vi "Create Arbitrary 111 Twin.vi"(10 "Additional Strain/twin (A)":dbl(slide) scale=0.0..10.0, 11 "Periodicity":i32[](array[numeric])=[3, 3]) -> (2 "# of extra cells needed for cubic":i32, 3 "AnBm Twin":T1={"Structure Name"="111 Twin, A6B1A4B1", "Lattice vector a"=[4.67354, 0.0, 0.0], "Lattice vector b"=[0.0, 8.0948, 0.0], "Lattice vector c"=[0.0, 0.0, 45.791158], "Atoms Array"=[{"Atom Name"="Cd", "Positions (Direct)"=[[0.0, 0.333334, 0.02083326728856693], [0.500001, 0.833335, 0.02083326728856693], [0.500001, 0.166667, 0.10416683644324957], [0.0, 0.666668, 0.10416683644324957], [0.0, 0.0, 0.18750008462334786], [0.500001, 0.500001, 0.18750008462334786], [0.0, 0.333334, 0.2708334092373685], [0.500001, 0.833335, 0.2708334092373685], [0.500001, 0.166667, 0.35416697839205113], [0.0, 0.666668, 0.35416697839205113], [0.0, 0.0, 0.4375002265721494], [0.500001, 0.500001, 0.4375002265721494], [0.500001, 0.166667, 0.5208335530060322], [0.0, 0.666668, 0.5208335530060322], [0.0, 0.0, 0.6041666821354701], [0.500001, 0.500001, 0.6041666821354701], [0.0, 0.333334, 0.6875000067494909], [0.500001, 0.833335, 0.6875000067494909], [0.500001, 0.166667, 0.7708335759041735], [0.0, 0.666668, 0.7708335759041735], [0.0, 0.0, 0.8541668240842718], [0.500001, 0.500001, 0.8541668240842718], [0.500001, 0.166667, 0.9375001505181546], [0.0, 0.666668, 0.9375001505181546]], "Positions (Cartesian)"=[[0.0, 2.6982720632, 0.9539794340669999], [2.3367746735400003, 6.745680158, 0.9539794340669999], [2.3367746735400003, 1.3491360316, 4.769920065932999], [0.0, 5.3965441264, 4.769920065932999], [0.0, 0.0, 8.585846000001093], [2.3367746735400003, 4.0474080948, 8.585846000001093], [0.0, 2.6982720632, 12.401775434067], [2.3367746735400003, 6.745680158, 12.401775434067], [2.3367746735400003, 1.3491360316, 16.217716065933], [0.0, 5.3965441264, 16.217716065933], [0.0, 0.0, 20.03364200000109], [2.3367746735400003, 4.0474080948, 20.03364200000109], [2.3367746735400003, 1.3491360316, 23.849571517400598], [0.0, 5.3965441264, 23.849571517400598], [0.0, 0.0, 27.66549200000109], [2.3367746735400003, 4.0474080948, 27.66549200000109], [0.0, 2.6982720632, 31.481421434067002], [2.3367746735400003, 6.745680158, 31.481421434067002], [2.3367746735400003, 1.3491360316, 35.297362065933], [0.0, 5.3965441264, 35.297362065933], [0.0, 0.0, 39.1132880000011], [2.3367746735400003, 4.0474080948, 39.1132880000011], [2.3367746735400003, 1.3491360316, 42.9292175174006], [0.0, 5.3965441264, 42.9292175174006]]}, {"Atom Name"="Te", "Positions (Direct)"=[[0.0, 0.0, 0.0], [0.500001, 0.500001, 0.0], [0.0, 0.333334, 0.08333356915468265], [0.500001, 0.833335, 0.08333356915468265], [0.500001, 0.166667, 0.16666681551492246], [0.0, 0.666668, 0.16666681551492246], [0.0, 0.0, 0.25000014194880155], [0.500001, 0.500001, 0.25000014194880155], [0.0, 0.333334, 0.3333337111034842], [0.500001, 0.833335, 0.3333337111034842], [0.500001, 0.166667, 0.41666695746372406], [0.0, 0.666668, 0.41666695746372406], [0.0, 0.0, 0.5000002838976031], [0.500001, 0.500001, 0.5000002838976031], [0.500001, 0.166667, 0.5833334130270448], [0.0, 0.666668, 0.5833334130270448], [0.0, 0.0, 0.6666667394609238], [0.500001, 0.500001, 0.6666667394609238], [0.0, 0.333334, 0.7500003086156065], [0.500001, 0.833335, 0.7500003086156065], [0.500001, 0.166667, 0.8333335549758464], [0.0, 0.666668, 0.8333335549758464], [0.0, 0.0, 0.9166668814097255], [0.500001, 0.500001, 0.9166668814097255]], "Positions (Cartesian)"=[[0.0, 0.0, 0.0], [2.3367746735400003, 4.0474080948, 0.0], [0.0, 2.6982720632, 3.815940631866], [2.3367746735400003, 6.745680158, 3.815940631866], [2.3367746735400003, 1.3491360316, 7.631866482600667], [0.0, 5.3965441264, 7.631866482600667], [0.0, 0.0, 11.447796], [2.3367746735400003, 4.0474080948, 11.447796], [0.0, 2.6982720632, 15.263736631866], [2.3367746735400003, 6.745680158, 15.263736631866], [2.3367746735400003, 1.3491360316, 19.079662482600668], [0.0, 5.3965441264, 19.079662482600668], [0.0, 0.0, 22.895592], [2.3367746735400003, 4.0474080948, 22.895592], [2.3367746735400003, 1.3491360316, 26.711512482600668], [0.0, 5.3965441264, 26.711512482600668], [0.0, 0.0, 30.527442], [2.3367746735400003, 4.0474080948, 30.527442], [0.0, 2.6982720632, 34.343382631866], [2.3367746735400003, 6.745680158, 34.343382631866], [2.3367746735400003, 1.3491360316, 38.15930848260067], [0.0, 5.3965441264, 38.15930848260067], [0.0, 0.0, 41.975238000000004], [2.3367746735400003, 4.0474080948, 41.975238000000004]]}], "# of atoms"=48})   [LabVIEW 2010]
uses:
  <vilib>/Analysis/baseanly.llb/A x Vector.vi
  <vilib>/Analysis/NI_AALBase.lvlib
panel:
  in  "Twins":T2(array[cluster])=[{"Structure Name"="111", "Lattice vector a"=[4.67354, 0.0, 0.0], "Lattice vector b"=[0.0, 8.0948, 0.0], "Lattice vector c"=[0.0, 0.0, 3.81592], "Atoms Array"=[{"Atom Name"="Cd", "Positions (Direct)"=[[0.500001, 0.166667, 0.24999987353], [0.0, 0.666668, 0.24999987353]], "Positions (Cartesian)"=[[2.3367746735400003, 1.3491360316, 0.9539795174005976], [0.0, 5.3965441264, 0.9539795174005976]]}, {"Atom Name"="Te", "Positions (Direct)"=[[0.0, 0.0, 0.0], [0.500001, 0.500001, 0.0]], "Positions (Cartesian)"=[[0.0, 0.0, 0.0], [2.3367746735400003, 4.0474080948, 0.0]]}], "# of atoms"=4}, {"Structure Name"="111", "Lattice vector a"=[4.67354, 0.0, 0.0], "Lattice vector b"=[0.0, 8.0948, 0.0], "Lattice vector c"=[0.0, 0.0, 3.81595], "Atoms Array"=[{"Atom Name"="Cd", "Positions (Direct)"=[[0.0, 0.333334, 0.250000402207], [0.500001, 0.833335, 0.250000402207]], "Positions (Cartesian)"=[[0.0, 2.6982720632, 0.9539890348018015], [2.3367746735400003, 6.745680158, 0.9539890348018015]]}, {"Atom Name"="Te", "Positions (Direct)"=[[0.500001, 0.166667, 2.49411e-06], [0.0, 0.666668, 2.49411e-06]], "Positions (Cartesian)"=[[2.3367746735400003, 1.3491360316, 9.5173990545e-06], [0.0, 5.3965441264, 9.5173990545e-06]]}], "# of atoms"=4}, {"Structure Name"="111", "Lattice vector a"=[4.67354, 0.0, 0.0], "Lattice vector b"=[0.0, 8.0948, 0.0], "Lattice vector c"=[0.0, 0.0, 3.81593], "Atoms Array"=[{"Atom Name"="Cd", "Positions (Direct)"=[[0.0, 0.0, 0.249999344852], [0.500001, 0.500001, 0.249999344852]], "Positions (Cartesian)"=[[0.0, 0.0, 0.9539800000010924], [2.3367746735400003, 4.0474080948, 0.9539800000010924]]}, {"Atom Name"="Te", "Positions (Direct)"=[[0.0, 0.333334, 1.2647e-07], [0.500001, 0.833335, 1.2647e-07]], "Positions (Cartesian)"=[[0.0, 2.6982720632, 4.826006671e-07], [2.3367746735400003, 6.745680158, 4.826006671e-07]]}], "# of atoms"=4}]
  in  "System Array 2":path[](array[path])=[path "D:/Ab-initio/Structures/2013-7-29 Base Structures/111 Bulk/11 Twin Components/POSCAR, 111, Left vnl down bulk", path "D:/Ab-initio/Structures/2013-7-29 Base Structures/111 Bulk/11 Twin Components/POSCAR, 111, Center vnl down bulk", path "D:/Ab-initio/Structures/2013-7-29 Base Structures/111 Bulk/11 Twin Components/POSCAR, 111, Right vnl down bulk", path "D:/Ab-initio/Structures/2013-7-29 Base Structures/111 Bulk/11 Twin Components/POSCAR, 111, Left vnl up bulk", path "D:/Ab-initio/Structures/2013-7-29 Base Structures/111 Bulk/11 Twin Components/POSCAR, 111, Center vnl up bulk", path "D:/Ab-initio/Structures/2013-7-29 Base Structures/111 Bulk/11 Twin Components/POSCAR, 111, Right vnl up bulk"]
  in  "Bulk":T2(array[cluster])=[{"Structure Name"="111", "Lattice vector a"=[4.67354, 0.0, 0.0], "Lattice vector b"=[0.0, 8.0948, 0.0], "Lattice vector c"=[0.0, 0.0, 3.815933], "Atoms Array"=[{"Atom Name"="Cd", "Positions (Direct)"=[[0.0, 0.333334, 0.249999], [0.500001, 0.833335, 0.249999]], "Positions (Cartesian)"=[[0.0, 2.6982720632, 0.9539794340669999], [2.3367746735400003, 6.745680158, 0.9539794340669999]]}, {"Atom Name"="Te", "Positions (Direct)"=[[0.0, 0.0, 0.0], [0.500001, 0.500001, 0.0]], "Positions (Cartesian)"=[[0.0, 0.0, 0.0], [2.3367746735400003, 4.0474080948, 0.0]]}], "# of atoms"=4}, {"Structure Name"="111", "Lattice vector a"=[4.67354, 0.0, 0.0], "Lattice vector b"=[0.0, 8.0948, 0.0], "Lattice vector c"=[0.0, 0.0, 3.815933], "Atoms Array"=[{"Atom Name"="Cd", "Positions (Direct)"=[[0.500001, 0.166667, 0.250001], [0.0, 0.666668, 0.250001]], "Positions (Cartesian)"=[[2.3367746735400003, 1.3491360316, 0.9539870659329999], [0.0, 5.3965441264, 0.9539870659329999]]}, {"Atom Name"="Te", "Positions (Direct)"=[[0.0, 0.333334, 2e-06], [0.500001, 0.833335, 2e-06]], "Positions (Cartesian)"=[[0.0, 2.6982720632, 7.631866e-06], [2.3367746735400003, 6.745680158, 7.631866e-06]]}], "# of atoms"=4}, {"Structure Name"="111", "Lattice vector a"=[4.67354, 0.0, 0.0], "Lattice vector b"=[0.0, 8.0948, 0.0], "Lattice vector c"=[0.0, 0.0, 3.81593], "Atoms Array"=[{"Atom Name"="Cd", "Positions (Direct)"=[[0.0, 0.0, 0.249999344852], [0.500001, 0.500001, 0.249999344852]], "Positions (Cartesian)"=[[0.0, 0.0, 0.9539800000010924], [2.3367746735400003, 4.0474080948, 0.9539800000010924]]}, {"Atom Name"="Te", "Positions (Direct)"=[[0.500001, 0.166667, 1.2647e-07], [0.0, 0.666668, 1.2647e-07]], "Positions (Cartesian)"=[[2.3367746735400003, 1.3491360316, 4.826006671e-07], [0.0, 5.3965441264, 4.826006671e-07]]}], "# of atoms"=4}]
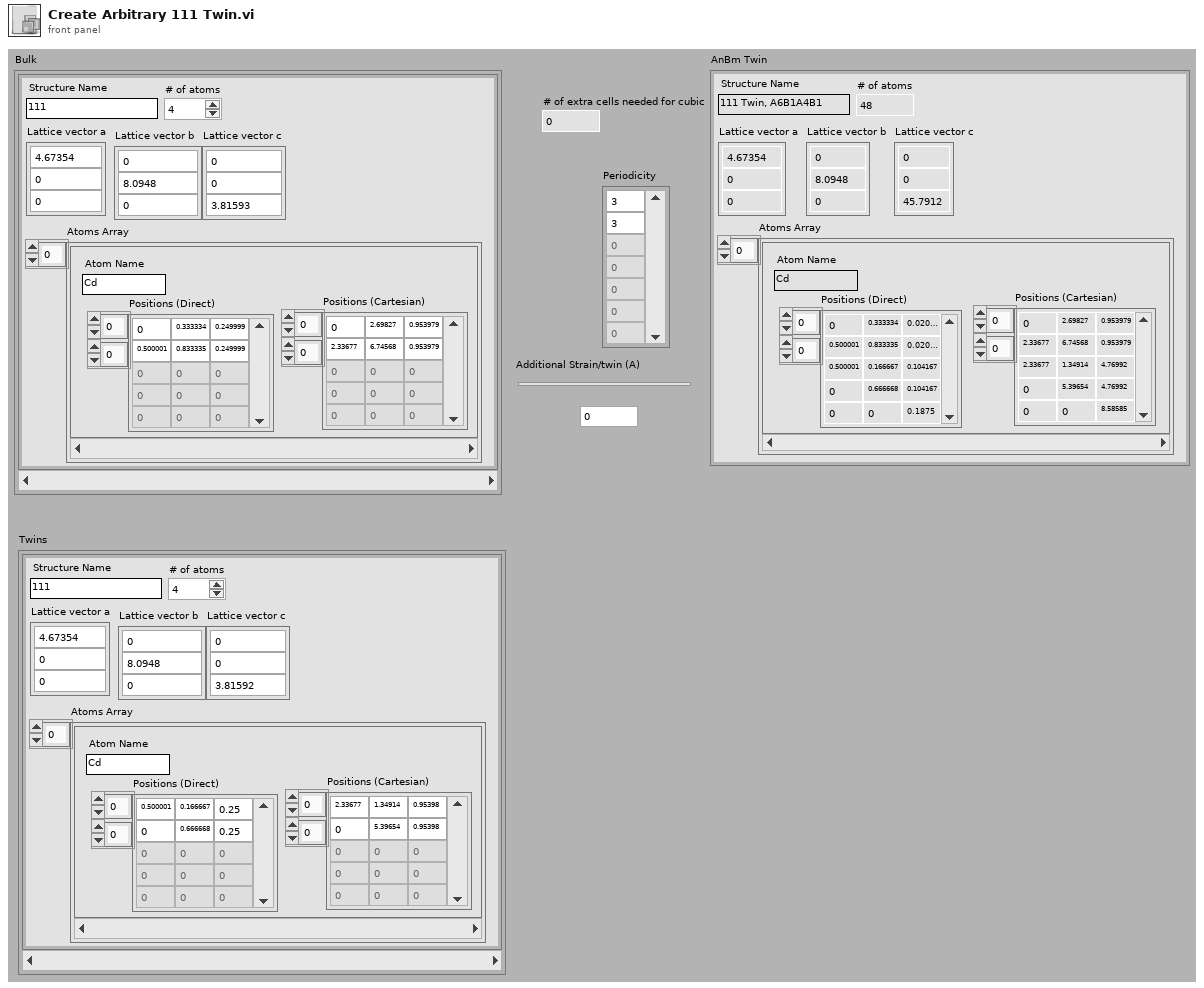
[diagram p1: front panel]
types:
  T1 = cluster{"Structure Name":string, "Lattice vector a":dbl[], "Lattice vector b":dbl[], "Lattice vector c":dbl[], "Atoms Array":cluster{"Atom Name":string, "Positions (Direct)":dbl[][], "Positions (Cartesian)":dbl[][]}[], "# of atoms":i32}
  T2 = cluster{"Structure Name":string, "Lattice vector a":dbl[], "Lattice vector b":dbl[], "Lattice vector c":dbl[], "Atoms Array":cluster{"Atom Name":string, "Positions (Direct)":dbl[][], "Positions (Cartesian)":dbl[][]}[], "# of atoms":i32}[]
  T3 = cluster{"Atom Name":string, "Positions (Direct)":dbl[][], "Positions (Cartesian)":dbl[][]}[]
  T4 = typedef "NI_Matrix.lvlib/RealMatrix.ctl" = dbl[][]
  T5 = cluster{"Atom Name":string, "Positions (Direct)":dbl[][], "Positions (Cartesian)":dbl[][]}
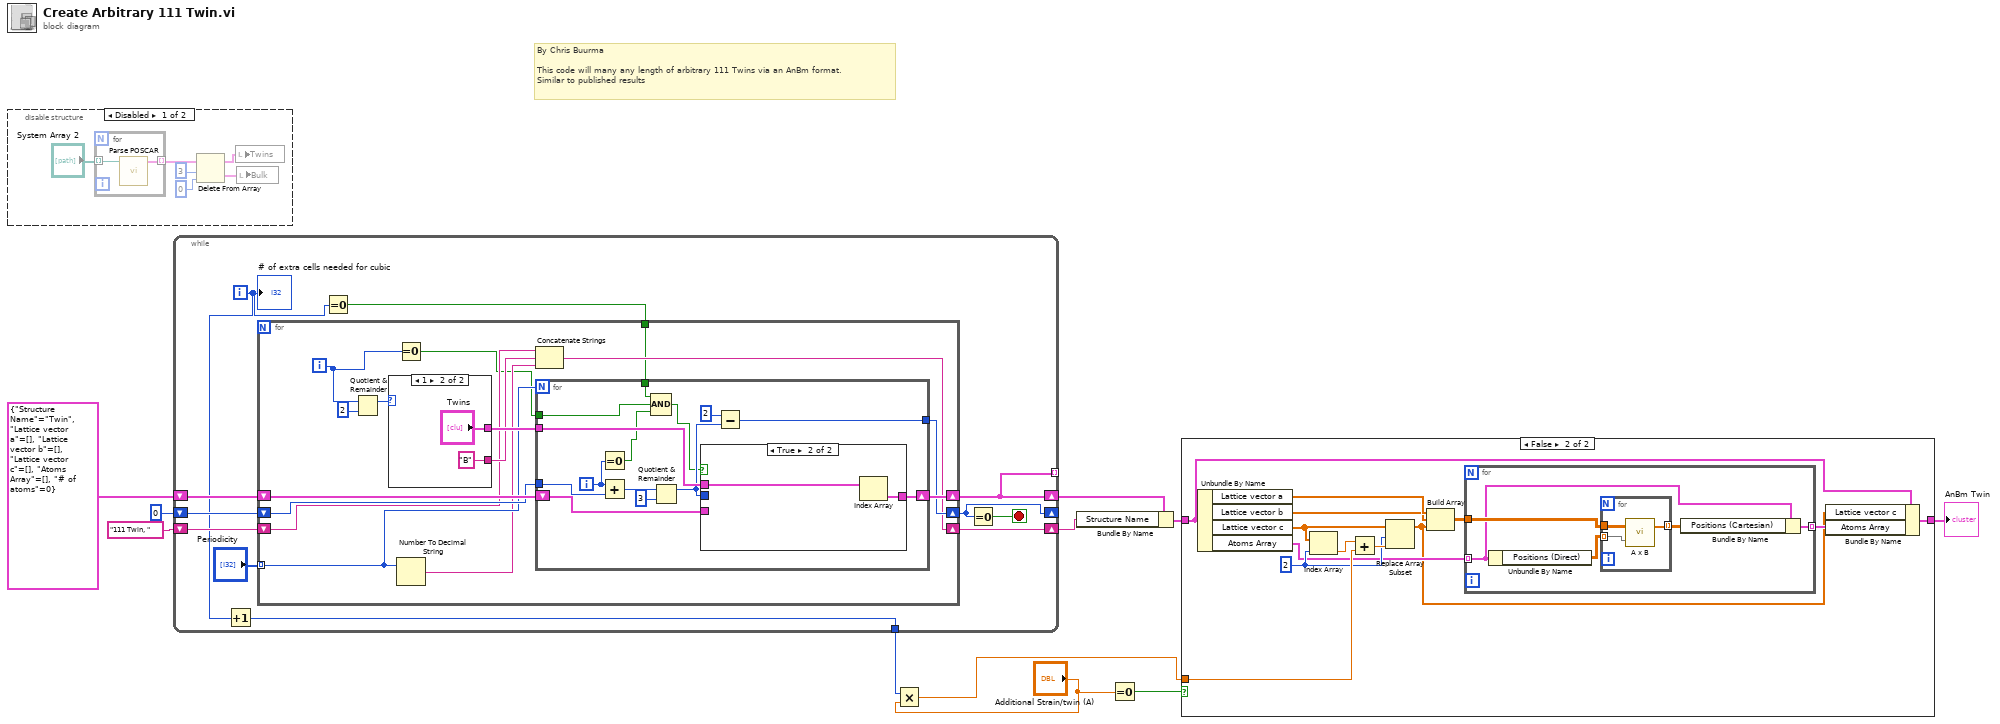
[diagram p0: block diagram]
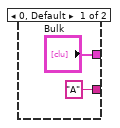
[diagram p2: hidden frame]
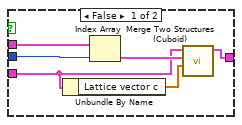
[diagram p3: hidden frame]
diagram:
  # "By Chris Buurma\n\nThis code will many any length of arbitrary 111 Twins via an AnBm format.\nSimilar to published results"
  n1 = disable-structure shown="Disabled" {
    frame Disabled {
      n2 = for {
        tunnel: [w19] -> w16 mode=indexing
        tunnel: "System Array 2" -> [w18] mode=indexing
        n3 = call "Parse POSCAR.vi"("POSCAR File"=w18) -> ("Structure"=w19:T1)  [unwired: 7 in, 3 out]
      }
      n4 = Delete From Array(array=w16, length=3, index=0) -> (deleted portion=w14:T2, array with subset deleted=w13:T2)
      n5 = local write "Twins"(w13) -> ()
      n6 = local write "Bulk"(w14) -> ()
    }
    frame Enabled {
    }
  }
  n7 = while {
    shift-right: [w26] -> w4
    shift-left: "111 Twin, " -> [w28]
    shift-right: [w23] -> w10
    shift-left: T1 {"Structure Name"="Twin", "Lattice vector a"=[], "Lattice vector b"=[], "Lattice vector c"=[], "Atoms Array"=[], "# of atoms"=0} ("Atomic Structure of 1 + 2 by T") -> [w29]
    shift-right: [w25] -> _
    shift-left: 0 -> [w27]
    tunnel: [w23] -> _ mode=indexing
    tunnel: [w20] -> w3
    i -> [w21]
    stop <- w24 stop-if-true
    n8 = Increment(x=w21) -> (x+1=w20:i32)
    n9 = Equal To 0?(x=w21) -> (x = 0?=w22:bool)
    n10 = for {
      tunnel: "Periodicity" -> [w37] mode=indexing
      shift-right: [w42] -> w23
      shift-left: w29 -> [w41]
      shift-right: [w40] -> w25
      shift-left: w27 -> [w39]
      shift-right: [w35] -> w26
      shift-left: w28 -> [w34]
      tunnel: w22 -> [w31]
      i -> [w33]
      n11 = Quotient & Remainder(x=w33, y=2) -> (x-y*floor(x/y)=w44:i32)  [unwired: 1 out]
      n12 = case shown="1" w44 {
        tunnel: ["Bulk" "Twins"] -> w43
        tunnel: ["A" ("string") "B" ("string")] -> w38
        frame 0, Default {
        }
        frame 1 {
        }
      }
      n13 = Equal To 0?(x=w33) -> (x = 0?=w32:bool)
      n14 = Number To Decimal String(number=w37) -> (decimal integer string=w36:string)  [unwired: 1 in]
      n15 = Concatenate Strings(w34, w38, w36) -> (w35:string)
      n16 = for {
        N: w37 -> [_]
        tunnel: w43 -> [w63]
        shift-right: [w61] -> w42
        shift-left: w41 -> [w60]
        tunnel: [w57] -> w40
        tunnel: w39 -> [w56]
        tunnel: w32 -> [w53]
        tunnel: w31 -> [w50]
        i -> [w54]
        n17 = Equal To 0?(x=w54) -> (x = 0?=w51:bool)
        n18 = Add(x=w54, y=w56) -> (x+y=w55:i32)
        n19 = Compound Arithmetic op=AND(w50, w53, w51) -> (w52:bool)
        n20 = Quotient & Remainder(x=w55, y=3) -> (x-y*floor(x/y)=w58:i32)  [unwired: 1 out]
        n21 = case shown="True" w52 {
          tunnel: w63 -> [w69 w71]
          tunnel: [w67 w70] -> w61
          tunnel: w60 -> [w66 _]
          tunnel: w58 -> [w64 _]
          frame False {
            n22 = Unbundle By Name(w66) -> ("Lattice vector c"=w65:dbl[])
            n23 = Index Array(array=w69, index=w64) -> (element=w68:T1)
            n24 = call "Merge Two Structures (Cuboid).vi"("Translation Vector (1 to 2)"=w65, "Atomic Structure 2"=w68, "Atomic Structure 1"=w66) -> ("Atomic Structure of 1 + 2 by T"=w67:T1)  [unwired: 8 in]
          }
          frame True {
            n25 = Index Array(array=w71) -> (element=w70:T1)  [unwired: 1 in]
          }
        }
        n26 = Subtract(x=2, y=w58) -> (x-y=w57:i32)
      }
    }
    n27 = Equal To 0?(x=w25) -> (x = 0?=w24:bool)
    "# of extra cells needed for cubic" <- w21
  }
  n28 = Multiply(x=w3, y="Additional Strain/twin (A)") -> (x*y=w1:dbl)
  n29 = Bundle By Name(cluster=w10, "Structure Name"=w4) -> (w9:T1)
  n30 = Equal To 0?(x="Additional Strain/twin (A)") -> (x = 0?=w7:bool)
  n31 = case shown="False" w7 {
    tunnel: w1 -> [_ w85]
    tunnel: w9 -> [w72 w74]
    tunnel: [w72 w73] -> w8
    frame True {
    }
    frame False {
      w82 = 2 ("index")
      n32 = Unbundle By Name(w74) -> ("Lattice vector a"=w81:dbl[], "Lattice vector b"=w80:dbl[], "Lattice vector c"=w79:dbl[], "Atoms Array"=w78:T3)
      n33 = Index Array(array=w79, index=w82) -> (element=w84:dbl)
      n34 = Add(x=w84, y=w85) -> (x+y=w83:dbl)
      n35 = Replace Array Subset(array=w79, new element=w83, index=w82) -> (w75:dbl[])
      n36 = Build Array(w81, w80, w75) -> (w77:T4)
      n37 = for {
        tunnel: w78 -> [w88] mode=indexing
        tunnel: w77 -> [w89]
        tunnel: [w86] -> w76 mode=indexing
        n38 = Unbundle By Name(w88) -> ("Positions (Direct)"=w90:dbl[][])
        n39 = for {
          tunnel: w90 -> [w93] mode=indexing
          tunnel: w89 -> [w92]
          tunnel: [w91] -> w87 mode=indexing
          n40 = call-poly <vilib>:"A x B.vi"("Vector"=w93, "A"=w92) -> ("A x Vector"=w91:dbl[])  [unwired: 1 out]
        }
        n41 = Bundle By Name(cluster=w88, "Positions (Cartesian)"=w87) -> (w86:T5)
      }
      n42 = Bundle By Name(cluster=w74, "Lattice vector c"=w75, "Atoms Array"=w76) -> (w73:T1)
    }
  }
  "AnBm Twin" <- w8
